vi "Emballage_BDD_NOMImprimante.vi"(8 "Error in":errorcluster caption="Error in (no error)") -> (0 "Error out":errorcluster, 3 "élément":string[](array[string]))   [LabVIEW 2020]
uses:
  Modules/FS/60_FS_Controles/60_FS_SetGet.ctl
  <vilib>/drjdpowell/SQLite Library/SQL Connection/Open (path).vi
  <vilib>/drjdpowell/SQLite Library/SQL Connection/Open (string).vi
  <vilib>/AdvancedString/Path To Command Line String.vi
  <vilib>/drjdpowell/SQLite Library/SQL Connection/Connection.lvclass
panel:
  out "Result Set":string[][](table) caption="Result Set (from first statement with results)"
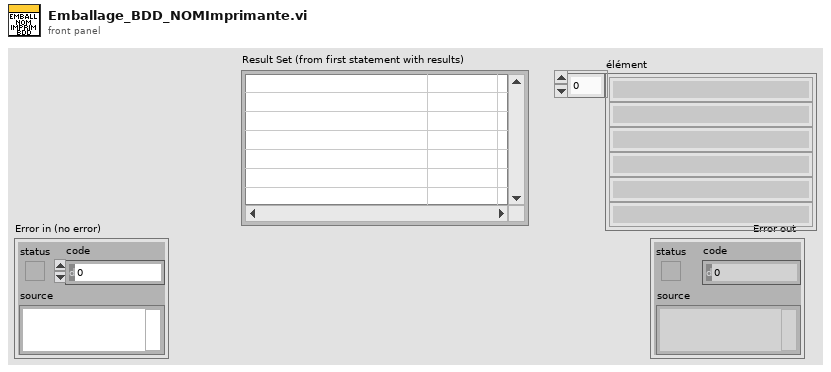
[diagram p1: front panel]
types:
  T1 = typedef "60_FS_SetGet.ctl" = enum16{"set", "get"}
  T2 = typedef "60_FS_CLT_Chemins.ctl" = cluster{"Racine_local":path, "Racine_reseau":path, "Racine_Support_Application":path, "Fichier_Journalisation":path, "Connexion_BDD_VSX":path, "Connexion_BDD_PLZ":path}
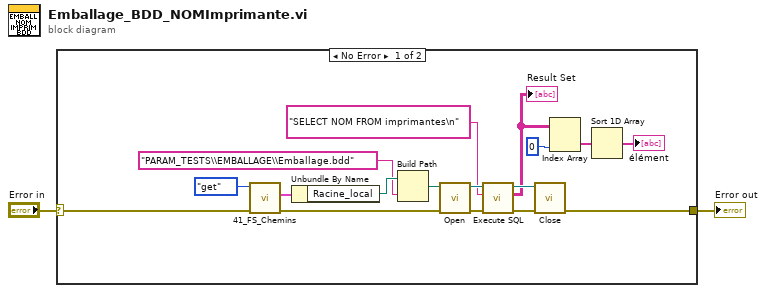
[diagram p0: block diagram]
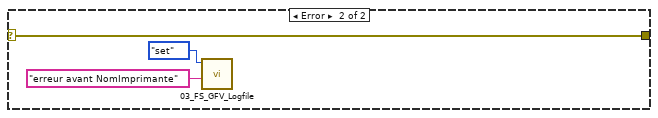
[diagram p2: hidden frame]
diagram:
  n1 = case shown="No Error" "Error in" {
    selector: "Error in" -> [w5 w20]
    tunnel: [w4 w20] -> w1
    frame No Error {
      n2 = call "41_FS_Chemins.vi"("error in (no error)"=w5, "SetGet"=60_FS_SetGet."get") -> ("error out"=w16:errorcluster, "CLT_Chemins_out"=w18:T2)  [unwired: 8 in]
      n3 = Unbundle By Name(w18) -> ("Racine_local"=w17:path)
      n4 = Build Path(base path=w17, name or relative path="PARAM_TESTS\\EMBALLAGE\\Emballage.bdd" ("nom ou chemin relatif")) -> (appended path=w10:path)
      n5 = call-poly <vilib>:"Open.vi"("error in (no error)"=w16, "db file"=w10) -> ("error out"=w15:errorcluster, "SQLite Connection"=w14:refnum<class "Connection.lvclass">)  [unwired: 8 in]
      n6 = call <vilib>:"Execute SQL.vi"("error in (no error)"=w15, "SQL"="SELECT NOM FROM imprimantes\n", "SQLite Connection in"=w14) -> ("error out"=w13:errorcluster, "Result Set"=w8:string[][], "SQLite Connection"=w12:refnum<class "Connection.lvclass">)  [unwired: 5 in, 1 out]
      "Result Set" <- w8
      n7 = call-dynamic "Close.vi"("error in (no error)"=w13, "SQLite Connection in"=w12) -> ("error out"=w4:errorcluster)  [unwired: 9 in]
      n8 = Index Array(array=w8, index (col)=0 ("indice (ligne)")) -> (element=w7:string[])  [unwired: 1 in]
      n9 = Sort 1D Array(array=w7) -> (sorted array=→"élément":string[])
    }
    frame Error {
      n10 = call "03_FS_GFV_Logfile.vi"("Chaîne"="erreur avant NomImprimante", "States"=60_FS_SetGet."set") -> ()  [unwired: 8 in, 2 out]
    }
  }
  "Error out" <- w1
